vi "Inst.Xeryon-Rotator.sendCommand.vi"(8 "error in (no error)":errorcluster, 9 "Value":dbl, 10 "Command":string, 11 "Inst.Xeryon-Rotator in":refnum<class "Inst.Xeryon-Rotator.lvclass">) -> (0 "error out":errorcluster, 3 "Inst.Xeryon-Rotator out":refnum<class "Inst.Xeryon-Rotator.lvclass">)   [LabVIEW 2019, in "Inst.Xeryon-Rotator.lvclass"]
uses:
  Inst.Xeryon-Rotator.lvclass
  Inst.Xeryon-Rotator.lvclass/Inst.Xeryon-Rotator.ctl
  Controller.LV/Controller.LV.lvclass
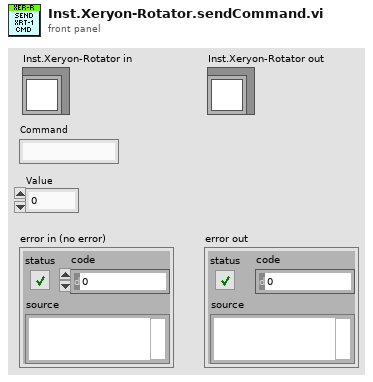
[diagram p1: front panel]
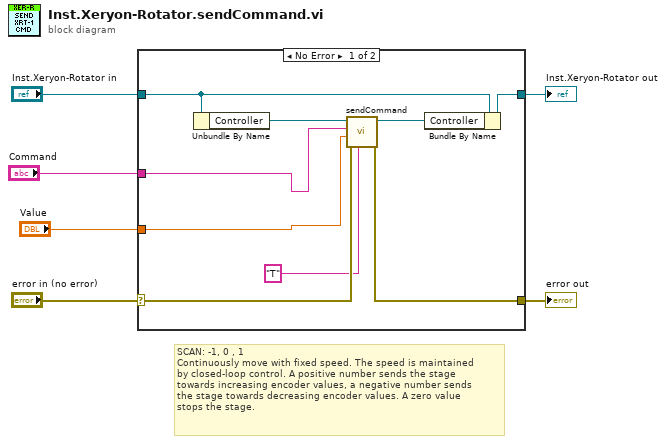
[diagram p0: block diagram]
diagram:
  # "SCAN: -1, 0 , 1\nContinuously move with fixed speed. The speed is maintained\nby closed-loop control. A positive number sends the stage\ntowards increasing encoder values, a negative number sends\nthe stage towards decreasing encoder values. A zero value\nstops the stage."
  n1 = case shown="No Error" "error in (no error)" {
    selector: "error in (no error)" -> [w12 w17]
    tunnel: "Inst.Xeryon-Rotator in" -> [w14 w16]
    tunnel: [w11 w17] -> w4
    tunnel: [w10 w16] -> w3
    tunnel: "Value" -> [w8 _]
    tunnel: "Command" -> [w7 _]
    frame No Error {
      n2 = Unbundle By Name(w14) -> ("Controller"=w15:refnum<class "Controller.LV.lvclass">)
      n3 = call-dynamic "sendCommand.vi"("Axis Letter"="T", "error in (no error)"=w12, "Value"=w8, "Command"=w7, "Controller in"=w15) -> ("error out"=w11:errorcluster, "Controller out"=w13:refnum<class "Controller.LV.lvclass">)  [unwired: 5 in]
      n4 = Bundle By Name(cluster=w14, "Controller"=w13) -> (w10:refnum<class "Inst.Xeryon-Rotator.lvclass">)
    }
    frame Error {
    }
  }
  "Inst.Xeryon-Rotator out" <- w3
  "error out" <- w4
